vi "display.vi"(8 "error in (no error)":errorcluster, 10 "CategoryList.lvclass":refnum<class "CategoryList.lvclass">, 11 "CategoryListUIAdapter in":refnum<class "CategoryListUIAdapter.lvclass">) -> (0 "error out":errorcluster, 3 "CategoryListUIAdapter out":refnum<class "CategoryListUIAdapter.lvclass">)   [LabVIEW 2020, in "CategoryListUIAdapter.lvclass"]
uses:
  CategoryListUIAdapter.lvclass
  CategoryList/CategoryList.lvclass
  <vilib>/Utility/miscctls.llb/LVRowAndColumnTypeDef.ctl
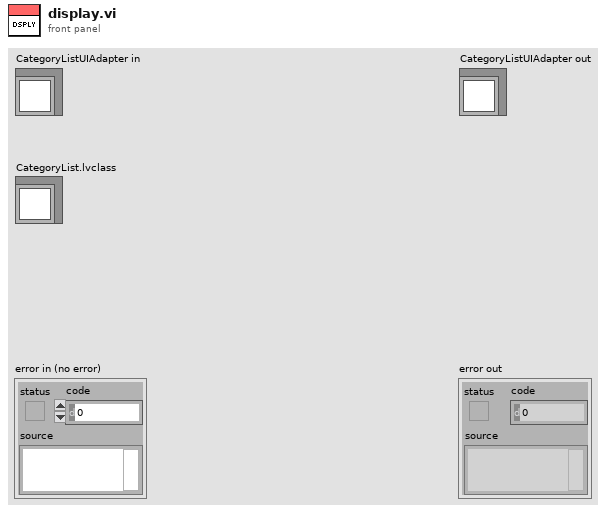
[diagram p1: front panel]
types:
  T1 = typedef "LVRowAndColumnTypeDef.ctl" = cluster{"Row":i32, "Column":i32}
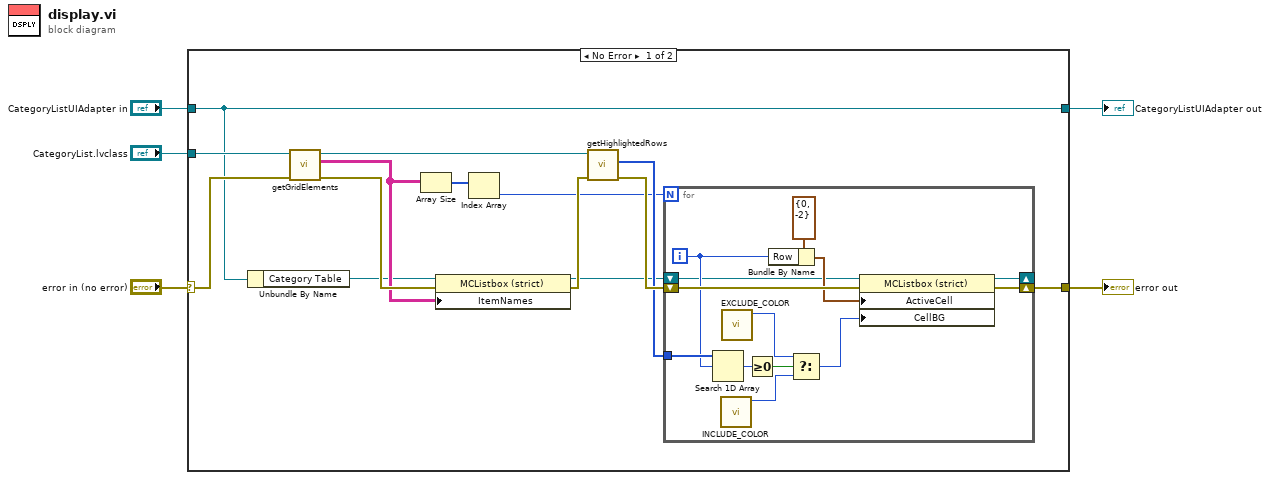
[diagram p0: block diagram]
diagram:
  n1 = case shown="No Error" "error in (no error)" {
    selector: "error in (no error)" -> [w11 w34]
    tunnel: [w10 w34] -> w4
    tunnel: [w8 w33] -> w2
    tunnel: "CategoryListUIAdapter in" -> [w8 w33]
    tunnel: "CategoryList.lvclass" -> [w12 _]
    frame No Error {
      n2 = Unbundle By Name(w8) -> ("Category Table"=w7:refnum<vi>)
      n3 = call "getGridElements.vi"("error in (no error)"=w11, "CategoryList in"=w12) -> ("error out"=w19:errorcluster, "Table Interface"=w15:string[][], "CategoryList out"=w9:refnum<class "CategoryList.lvclass">)  [unwired: 7 in]
      n4 = Array Size(array=w15) -> (size(s)=w14:i32[])
      n5 = property on="Property Node" class="MCListbox (strict)"(reference=w7, error in=w19, "ItemNames"=w15) -> (reference out=w6:refnum<vi>, error out=w18:errorcluster)
      n6 = Index Array(array=w14) -> (element=w13:i32)  [unwired: 1 in]
      n7 = call "getHighlightedRows.vi"("error in (no error)"=w18, "CategoryList in"=w9) -> ("error out"=w17:errorcluster, "Highlighted Rows"=w16:i32[])  [unwired: 7 in, 1 out]
      n8 = for {
        N: w13 -> [_]
        shift-right: [w31] -> w10
        shift-left: w17 -> [w32]
        tunnel: w16 -> [w27]
        shift-right: [w22] -> _
        shift-left: w6 -> [w23]
        i -> [w26]
        n9 = Search 1D Array(1D array=w27, element=w26) -> (index of element=w25:i32)  [unwired: 1 in]
        n10 = call "INCLUDE_COLOR.vi"() -> ("Color Box"=w20:u32)  [unwired: 11 in]
        n11 = call "EXCLUDE_COLOR.vi"() -> ("Color Box"=w21:u32)  [unwired: 11 in]
        n12 = Greater Or Equal To 0?(x=w25) -> (x >= 0?=w24:bool)
        n13 = Bundle By Name(cluster=T1 {"Row"=0, "Column"=-2} ("Active Cell:Active Cell"), "Row"=w26) -> (w28:T1)
        n14 = Select(t=w21, s=w24, f=w20) -> (s? t:f=w29:u32)
        n15 = property on="Property Node" class="MCListbox (strict)"(reference=w23, error in=w32, "ActiveCell"=w28, "CellBG"=w29) -> (reference out=w22:refnum<vi>, error out=w31:errorcluster)
      }
    }
    frame Error {
    }
  }
  "error out" <- w4
  "CategoryListUIAdapter out" <- w2
